vi "ScanDelayGetScannerFrequency.vi"(8 "error in (no error)":errorcluster, 9 "wait":u32=10, 11 "VISA resource name in":refnum<visa-resource-name>) -> (0 "error out":errorcluster, 2 "value":dbl, 3 "VISA resource name out":refnum<visa-resource-name>)   [LabVIEW 2018]
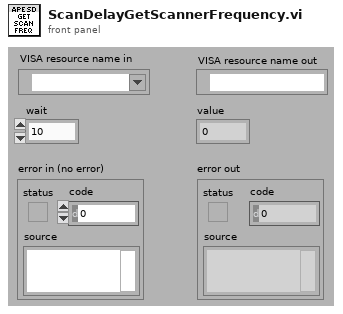
[diagram p1: front panel]
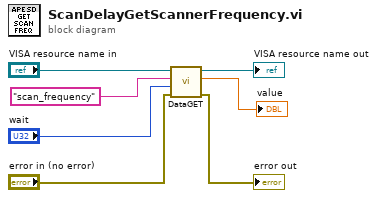
[diagram p0: block diagram]
diagram:
  n1 = call "DataGET.vi"("error in"="error in (no error)", "wait"="wait", "parameter"="scan_frequency", "VISA resource name"="VISA resource name in") -> ("error out"=→"error out":errorcluster, "value"=→"value":dbl, "VISA resource name out"=→"VISA resource name out":refnum<visa-resource-name>)  [unwired: 4 in]
